vi "Send Frame.vi"(8 "Error In":errorcluster, 10 "Frame":u32[][](array[colorbox]), 11 "Display In":refnum<class "Display.lvclass">) -> (0 "Error Out":errorcluster, 3 "Display Out":refnum<class "Display.lvclass">)   [LabVIEW 2019, in "Display.lvclass"]
uses:
  Display.lvclass
  Shared/Public/Controls/Neopixel FIFO Command.ctl
  Shared/Neopixel Shared.lvlib
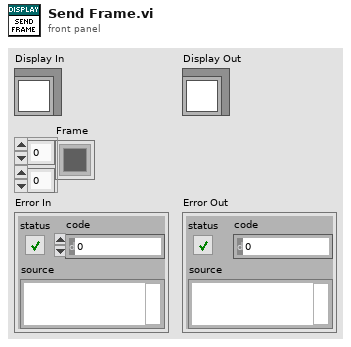
[diagram p1: front panel]
types:
  T1 = typedef "Neopixel Shared.lvlib/Neopixel FIFO Command.ctl" = enum8{"Set Number Of Neopixels", "Update Frame"}
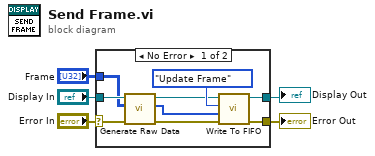
[diagram p0: block diagram]
diagram:
  n1 = case shown="No Error" "Error In" {
    selector: "Error In" -> [w11 w15]
    tunnel: "Display In" -> [w10 w16]
    tunnel: [w14 w15] -> w3
    tunnel: [w13 w16] -> w2
    tunnel: "Frame" -> [w9 _]
    frame No Error {
      n2 = call "Generate Raw Data.vi"("Error In"=w11, "Matrix"=w9, "Display In"=w10) -> ("Error Out"=w7:errorcluster, "Raw Data"=w8:u8[], "Display Out"=w6:refnum<class "Display.lvclass">)  [unwired: 6 in]
      n3 = call "Write To FIFO.vi"("Error In"=w7, "Data"=w8, "Command"=Neopixel_FIFO_Command."Update Frame", "Display In"=w6) -> ("Error Out"=w14:errorcluster, "Display Out"=w13:refnum<class "Display.lvclass">)  [unwired: 6 in]
    }
    frame Error {
    }
  }
  "Error Out" <- w3
  "Display Out" <- w2
